vi "saveFreqSweep.vi"(9 "f-res, Hz":dbl, 10 "Frequency Scan":cluster{i32[], "Best Gaussian Fit":dbl[]}[](array[cluster]), 11 "file path (dialog if empty)":path) -> ()   [LabVIEW 2011]
uses:
  <vilib>/Utility/file.llb/Write To Spreadsheet File (DBL).vi
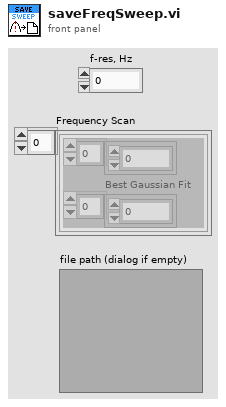
[diagram p1: front panel]
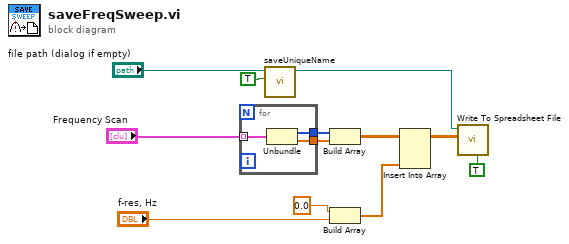
[diagram p0: block diagram]
diagram:
  n1 = for {
    tunnel: "Frequency Scan" -> [w15] mode=indexing
    tunnel: [w14] -> w11
    tunnel: [w13] -> w12
    n2 = Unbundle(w15) -> (w14:i32[], "Best Gaussian Fit"=w13:dbl[])
  }
  n3 = call "saveUniqueName.vi"("Check existence before modifying path"=TRUE, "path"="file path (dialog if empty)") -> ("unique path"=w6:path)  [unwired: 8 in, 1 out]
  n4 = Build Array(w11, w12) -> (w3:dbl[][])
  n5 = Build Array(0.0 ("element"), "f-res, Hz") -> (w2:dbl[])
  n6 = Insert Into Array(array=w3, new element=w2) -> (w1:dbl[][])  [unwired: 2 in]
  n7 = call-poly <vilib>:"Write To Spreadsheet File.vi"("transpose? (no:F)"=TRUE, "2D data"=w1, "file path (dialog if empty)"=w6) -> ()  [unwired: 5 in, 1 out]
